vi "basic.vi"() -> ()   [LabVIEW 2019]
panel:
  in  "Version":u8(ring) items=["Li-Ion"=1, "Ni-MH"=2]
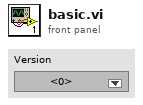
[diagram p1: front panel]
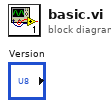
[diagram p0: block diagram]
diagram:
